vi "cameraTempControllerBackEnd.vi"(8 "error in (no error)":errorcluster, 11 "CameraTempController":refnum<class "CameraTempController.lvclass">) -> (0 "error out":errorcluster, 3 "CameraTempController out":refnum<class "CameraTempController.lvclass">)   [LabVIEW 2011, in "Hardware.lvlib" / "Channels.lvlib" / "CameraTempController.lvclass"]
uses:
  CameraTempController.lvclass
panel:
  in  "tempControllerBackEndEvents":T1
  in  "tempControllerFrontEndEvents":T2
  out "Cooling":bool=TRUE
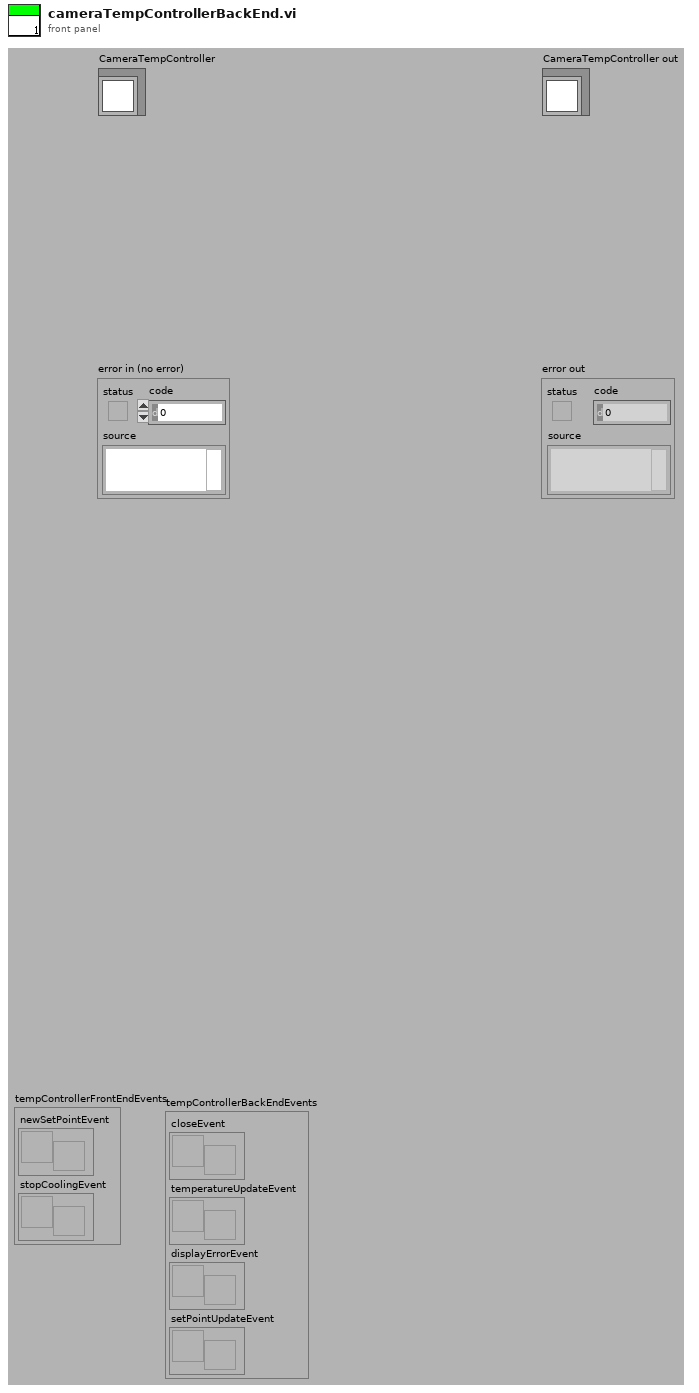
[diagram p1: front panel]
types:
  T1 = cluster{"closeEvent":refnum<user-event>, "temperatureUpdateEvent":refnum<user-event>, "displayErrorEvent":refnum<user-event>, "setPointUpdateEvent":refnum<user-event>}
  T2 = cluster{"newSetPointEvent":refnum<user-event>, "stopCoolingEvent":refnum<user-event>}
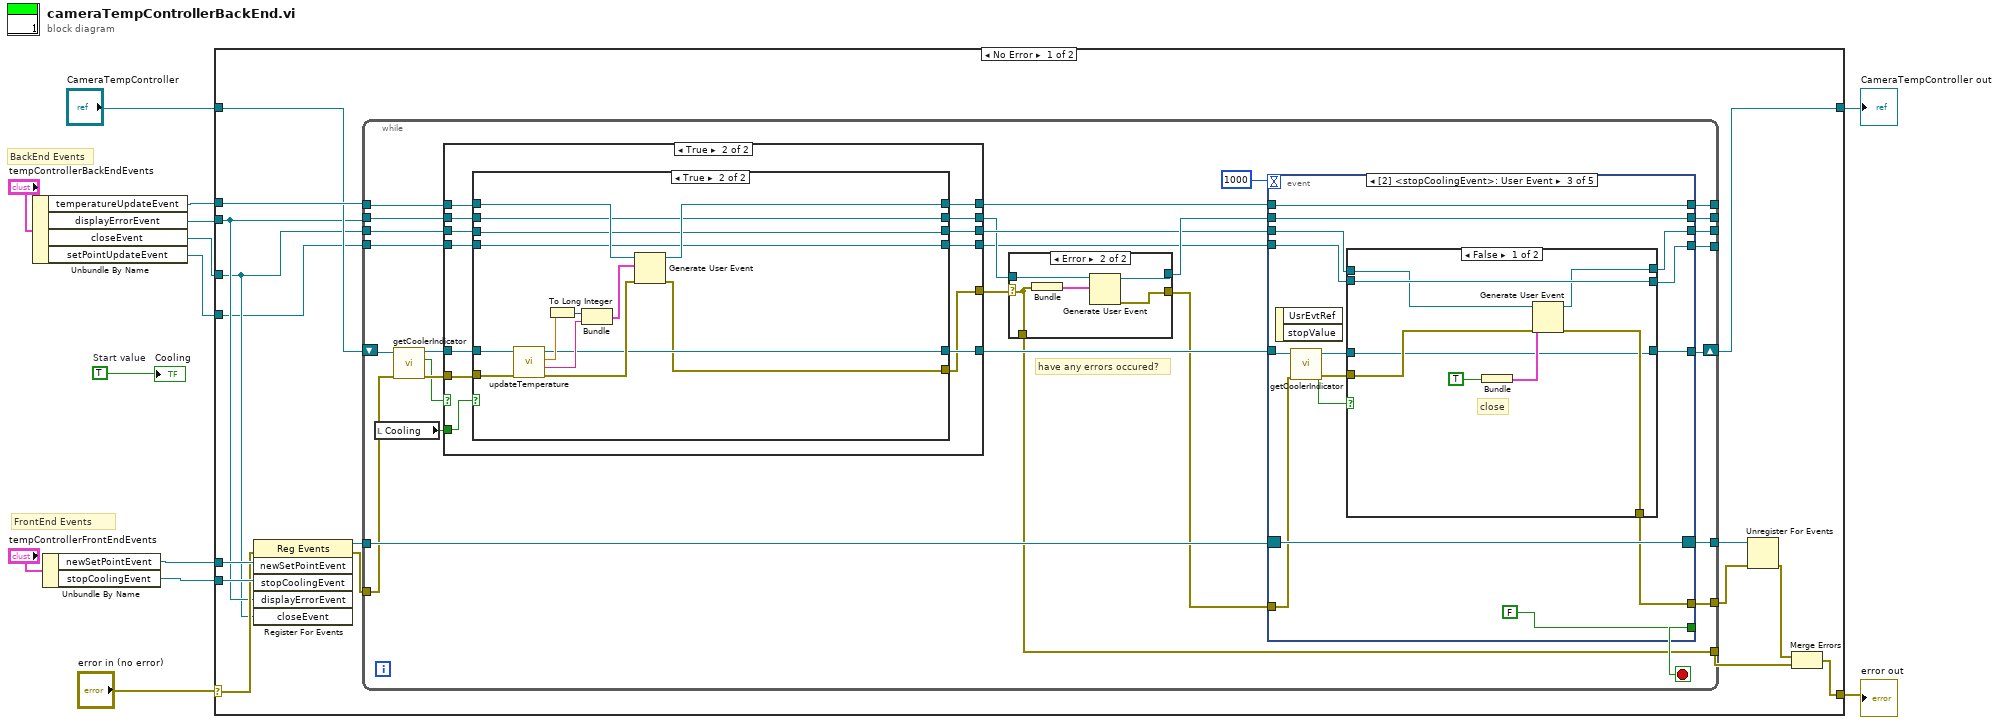
[diagram p0: block diagram]
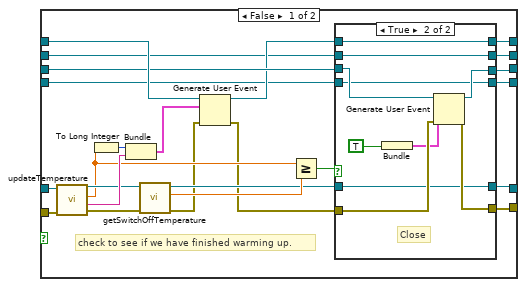
[diagram p3: hidden frame]
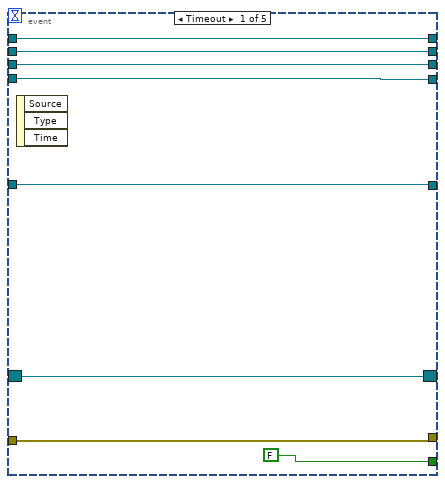
[diagram p6: hidden frame]
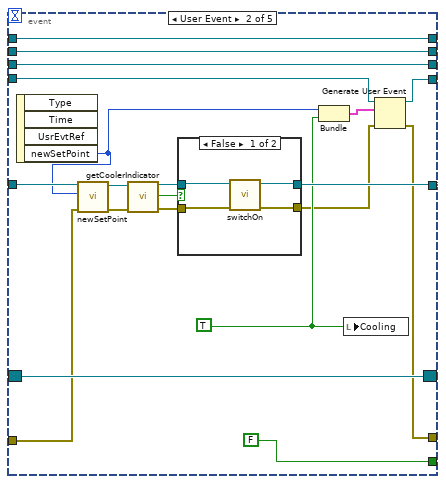
[diagram p7: hidden frame]
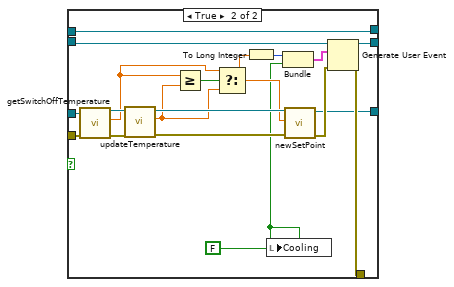
[diagram p9: hidden frame]
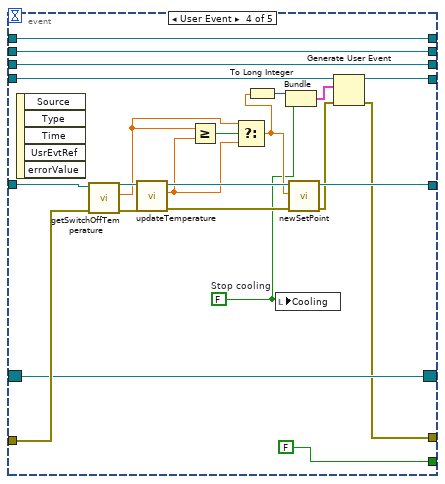
[diagram p10: hidden frame]
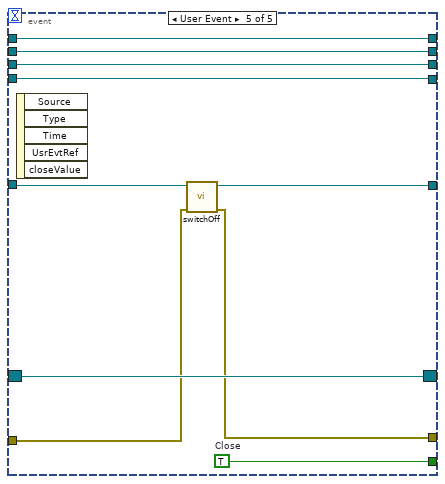
[diagram p11: hidden frame]
diagram:
  w9 = TRUE  # Start value
  # "FrontEnd Events"
  # "BackEnd Events"
  n1 = Unbundle By Name("tempControllerBackEndEvents") -> ("temperatureUpdateEvent"=w4:refnum<user-event>, "displayErrorEvent"=w3:refnum<user-event>, "closeEvent"=w2:refnum<user-event>, "setPointUpdateEvent"=w1:refnum<user-event>)
  n2 = Unbundle By Name("tempControllerFrontEndEvents") -> ("newSetPointEvent"=w5:refnum<user-event>, "stopCoolingEvent"=w6:refnum<user-event>)
  n3 = case shown="No Error" "error in (no error)" {
    selector: "error in (no error)" -> [w27 w249]
    tunnel: [w16 w249] -> w12
    tunnel: [w22 w248] -> w10
    tunnel: "CameraTempController" -> [w24 w248]
    tunnel: w4 -> [w26 _]
    tunnel: w3 -> [w21 _]
    tunnel: w2 -> [w19 _]
    tunnel: w5 -> [w29 _]
    tunnel: w6 -> [w28 _]
    tunnel: w1 -> [w15 _]
    frame No Error {
      n4 = register-events(error in=w27, w29, w28, w21, w19) -> (reference out=w25:refnum<event-registration>, error out=w20:errorcluster)  [unwired: 1 in]
      n5 = while {
        tunnel: w26 -> [w54]
        tunnel: w21 -> [w42]
        tunnel: w19 -> [w44]
        tunnel: w25 -> [w58]
        tunnel: w20 -> [w33]
        tunnel: [w57] -> _
        tunnel: [w56] -> _
        tunnel: [w55] -> w23
        shift-right: [w50] -> w22
        shift-left: w24 -> [w34]
        tunnel: [w52] -> _
        tunnel: [w49] -> w14
        tunnel: [w39] -> w17
        tunnel: w15 -> [w38]
        tunnel: [w36] -> _
        stop <- w40 stop-if-true
        # "have any errors occured?"
        n6 = local read "Cooling"() -> (w45:bool)
        n7 = call-dynamic "getCoolerIndicator.vi"("error in (no error)"=w33, "CameraTempController.lvclass in"=w34) -> ("error out"=w32:errorcluster, "Cooler"=w31:bool, "CameraTempController.lvclass out"=w35:refnum<class "CameraTempController.lvclass">)  [unwired: 7 in]
        n8 = case shown="True" w31 {
          tunnel: w54 -> [w64 w77]
          tunnel: [w64 w76] -> w53
          tunnel: [w61 w75] -> w51
          tunnel: [w59 w74] -> w48
          tunnel: w45 -> [_ w73]
          tunnel: w44 -> [w60 w72]
          tunnel: [w60 w71] -> w43
          tunnel: w42 -> [w62 w70]
          tunnel: [w62 w69] -> w41
          tunnel: w38 -> [w63 w68]
          tunnel: [w63 w67] -> w37
          tunnel: w35 -> [w61 w66]
          tunnel: w32 -> [w59 w65]
          frame False {
          }
          frame True {
            n9 = case shown="True" w73 {
              tunnel: w66 -> [w98 w127]
              tunnel: w77 -> [w99 w126]
              tunnel: [w84 w125] -> w76
              tunnel: w65 -> [w97 w124]
              tunnel: [w86 w123] -> w75
              tunnel: [w87 w122] -> w74
              tunnel: w72 -> [w88 w121]
              tunnel: [w85 w121] -> w71
              tunnel: w70 -> [w82 w120]
              tunnel: [w81 w120] -> w69
              tunnel: w68 -> [w80 w119]
              tunnel: [w79 w119] -> w67
              frame False {
                # "check to see if we have finished warming up."
                n10 = call-dynamic "updateTemperature.vi"("error in (no error)"=w97, "CameraTempController in"=w98) -> ("error out"=w95:errorcluster, "Status"=w101:string, "updateTemperature"=w94:dbl, "CameraTempController out"=w96:refnum<class "CameraTempController.lvclass">)  [unwired: 6 in]
                n11 = To Long Integer(number=w94) -> (32bit integer=w78:i32)
                n12 = Bundle(w78, "Status"=w101) -> (w100:cluster{i32, "Status":string})  [unwired: 1 in]
                n13 = call-dynamic "getSwitchOffTemperature.vi"("error in (no error)"=w95, "CameraTempController in"=w96) -> ("error out"=w90:errorcluster, "Switch Off Temperature"=w93:dbl, "CameraTempController out"=w91:refnum<class "CameraTempController.lvclass">)  [unwired: 7 in]
                n14 = Generate User Event(user event=w99, event data cluster=w100, error in=w90) -> (user event out=w83:refnum<user-event>, error out=w89:errorcluster)
                n15 = Greater Or Equal?(x=w94, y=w93) -> (x >= y?=w92:bool)
                n16 = case shown="True" w92 {
                  tunnel: w91 -> [w107 w114]
                  tunnel: w89 -> [w106 w116]
                  tunnel: w88 -> [w105 w117]
                  tunnel: [w106 w115] -> w87
                  tunnel: [w107 w114] -> w86
                  tunnel: [w105 w113] -> w85
                  tunnel: [w103 w110] -> w84
                  tunnel: w83 -> [w103 w110]
                  tunnel: w82 -> [w104 w109]
                  tunnel: [w104 w109] -> w81
                  tunnel: [w102 w108] -> w79
                  tunnel: w80 -> [w102 w108]
                  frame False {
                  }
                  frame True {
                    # "Close"
                    n17 = Bundle(TRUE) -> (w111:cluster{bool})  [unwired: 1 in]
                    n18 = Generate User Event(user event=w117, event data cluster=w111, error in=w116) -> (user event out=w113:refnum<user-event>, error out=w115:errorcluster)
                  }
                }
              }
              frame True {
                n19 = call-dynamic "updateTemperature.vi"("error in (no error)"=w124, "CameraTempController in"=w127) -> ("error out"=w128:errorcluster, "Status"=w130:string, "updateTemperature"=w131:dbl, "CameraTempController out"=w123:refnum<class "CameraTempController.lvclass">)  [unwired: 6 in]
                n20 = To Long Integer(number=w131) -> (32bit integer=w118:i32)
                n21 = Bundle(w118, "Status"=w130) -> (w129:cluster{i32, "Status":string})  [unwired: 1 in]
                n22 = Generate User Event(user event=w126, event data cluster=w129, error in=w128) -> (user event out=w125:refnum<user-event>, error out=w122:errorcluster)
              }
            }
          }
        }
        n23 = case shown="Error" w48 {
          selector: w48 -> [w132 w134]
          tunnel: [w132 w136] -> w47
          tunnel: w41 -> [w133 w138]
          tunnel: [w133 w135] -> w46
          tunnel: [w132 w134] -> w39
          frame No Error {
          }
          frame Error {
            n24 = Bundle("error IO"=w134) -> (w137:cluster{"error IO":errorcluster})  [unwired: 1 in]
            n25 = Generate User Event(user event=w138, event data cluster=w137) -> (user event out=w135:refnum<user-event>, error out=w136:errorcluster)  [unwired: 1 in]
          }
        }
        n26 = event shown="[2] <stopCoolingEvent>: User Event" {
          selector: w58 -> [w141 w163 w185 w232 w246]
          dyn-events: [w141 w163 w185 w232 w246] -> w55
          timeout: 1000 -> [_ _ _ _ _]
          tunnel: w53 -> [w146 w166 w187 w237 w245]
          tunnel: w46 -> [w145 w165 w186 w236 w244]
          tunnel: w43 -> [w144 w164 w175 w235 w243]
          tunnel: w47 -> [w142 w162 w180 w233 w240]
          tunnel: [w146 w166 w187 w237 w245] -> w52
          tunnel: [w145 w165 w186 w236 w244] -> w57
          tunnel: [w144 w164 w174 w235 w243] -> w56
          tunnel: [w143 w156 w173 w231 w241] -> w50
          tunnel: [w142 w147 w181 w219 w239] -> w49
          tunnel: w51 -> [w143 w155 w179 w234 w242]
          tunnel: [FALSE FALSE FALSE FALSE w247] -> w40
          tunnel: w37 -> [w139 w153 w183 w222 w238]
          tunnel: [w139 w152 w182 w221 w238] -> w36
          event Timeout {
            n27 = event-data() -> ()  [unwired: 1 in, 3 out]
          }
          event User Event {
            w149 = TRUE
            n28 = event-data() -> ("newSetPoint"=w151:i32)  [unwired: 1 in, 3 out]
            n29 = call-dynamic "newSetPoint.vi"("error in (no error)"=w162, "setTemperature"=w151, "CameraTempController in"=w155) -> ("error out"=w160:errorcluster, "CameraTempController out"=w161:refnum<class "CameraTempController.lvclass">)  [unwired: 7 in]
            n30 = call-dynamic "getCoolerIndicator.vi"("error in (no error)"=w160, "CameraTempController.lvclass in"=w161) -> ("error out"=w157:errorcluster, "Cooler"=w159:bool, "CameraTempController.lvclass out"=w158:refnum<class "CameraTempController.lvclass">)  [unwired: 7 in]
            n31 = case shown="False" w159 {
              tunnel: w158 -> [w170 w172]
              tunnel: w157 -> [w169 w171]
              tunnel: [w167 w172] -> w156
              tunnel: [w168 w171] -> w148
              frame False {
                n32 = call-dynamic "switchOn.vi"("error in (no error)"=w169, "CameraTempController in"=w170) -> ("error out"=w168:errorcluster, "CameraTempController out"=w167:refnum<class "CameraTempController.lvclass">)  [unwired: 8 in]
              }
              frame True {
              }
            }
            n33 = Bundle("newSetPoint"=w151, w149) -> (w150:cluster{"newSetPoint":i32, bool})  [unwired: 1 in]
            n34 = local write "Cooling"(w149) -> ()
            n35 = Generate User Event(user event=w153, event data cluster=w150, error in=w148) -> (user event out=w152:refnum<user-event>, error out=w147:errorcluster)
          }
          event User Event {
            n36 = event-data() -> ()  [unwired: 1 in, 2 out]
            n37 = call-dynamic "getCoolerIndicator.vi"("error in (no error)"=w180, "CameraTempController.lvclass in"=w179) -> ("error out"=w176:errorcluster, "Cooler"=w178:bool, "CameraTempController.lvclass out"=w177:refnum<class "CameraTempController.lvclass">)  [unwired: 7 in]
            n38 = case shown="False" w178 {
              tunnel: w183 -> [w193 w207]
              tunnel: [w193 w206] -> w182
              tunnel: [w189 w203] -> w181
              tunnel: w177 -> [w188 w199]
              tunnel: w176 -> [w190 w198]
              tunnel: w175 -> [w192 w197]
              tunnel: [w191 w197] -> w174
              tunnel: [w188 w196] -> w173
              frame False {
                # "close"
                n39 = Bundle(TRUE) -> (w194:cluster{bool})  [unwired: 1 in]
                n40 = Generate User Event(user event=w192, event data cluster=w194, error in=w190) -> (user event out=w191:refnum<user-event>, error out=w189:errorcluster)
              }
              frame True {
                w201 = FALSE
                n41 = call-dynamic "getSwitchOffTemperature.vi"("error in (no error)"=w198, "CameraTempController in"=w199) -> ("error out"=w211:errorcluster, "Switch Off Temperature"=w209:dbl, "CameraTempController out"=w212:refnum<class "CameraTempController.lvclass">)  [unwired: 7 in]
                n42 = call-dynamic "updateTemperature.vi"("error in (no error)"=w211, "CameraTempController in"=w212) -> ("error out"=w214:errorcluster, "updateTemperature"=w208:dbl, "CameraTempController out"=w213:refnum<class "CameraTempController.lvclass">)  [unwired: 6 in, 1 out]
                n43 = Greater Or Equal?(x=w209, y=w208) -> (x >= y?=w210:bool)
                n44 = Select(t=w209, s=w210, f=w208) -> (s? t:f=w202:dbl)
                n45 = To Long Integer(number=w202) -> (32bit integer=w200:i32)
                n46 = local write "Cooling"(w201) -> ()
                n47 = Bundle(w200, w201) -> (w205:cluster{i32, bool})  [unwired: 1 in]
                n48 = call-dynamic "newSetPoint.vi"("error in (no error)"=w214, "setTemperature"=w202, "CameraTempController in"=w213) -> ("error out"=w204:errorcluster, "CameraTempController out"=w196:refnum<class "CameraTempController.lvclass">)  [unwired: 7 in]
                n49 = Generate User Event(user event=w207, event data cluster=w205, error in=w204) -> (user event out=w206:refnum<user-event>, error out=w203:errorcluster)
              }
            }
          }
          event User Event {
            w216 = FALSE  # Stop cooling
            n50 = event-data() -> ()  [unwired: 1 in, 5 out]
            n51 = call-dynamic "getSwitchOffTemperature.vi"("error in (no error)"=w233, "CameraTempController in"=w234) -> ("error out"=w227:errorcluster, "Switch Off Temperature"=w225:dbl, "CameraTempController out"=w228:refnum<class "CameraTempController.lvclass">)  [unwired: 7 in]
            n52 = call-dynamic "updateTemperature.vi"("error in (no error)"=w227, "CameraTempController in"=w228) -> ("error out"=w230:errorcluster, "updateTemperature"=w224:dbl, "CameraTempController out"=w229:refnum<class "CameraTempController.lvclass">)  [unwired: 6 in, 1 out]
            n53 = Greater Or Equal?(x=w225, y=w224) -> (x >= y?=w226:bool)
            n54 = Select(t=w225, s=w226, f=w224) -> (s? t:f=w217:dbl)
            n55 = To Long Integer(number=w217) -> (32bit integer=w215:i32)
            n56 = local write "Cooling"(w216) -> ()
            n57 = Bundle(w215, "Stop cooling"=w216) -> (w218:cluster{i32, "Stop cooling":bool})  [unwired: 1 in]
            n58 = call-dynamic "newSetPoint.vi"("error in (no error)"=w230, "setTemperature"=w217, "CameraTempController in"=w229) -> ("error out"=w220:errorcluster, "CameraTempController out"=w231:refnum<class "CameraTempController.lvclass">)  [unwired: 7 in]
            n59 = Generate User Event(user event=w222, event data cluster=w218, error in=w220) -> (user event out=w221:refnum<user-event>, error out=w219:errorcluster)
          }
          event User Event {
            w247 = TRUE  # Close
            n60 = event-data() -> ()  [unwired: 1 in, 5 out]
            n61 = call-dynamic "switchOff.vi"("error in (no error)"=w240, "CameraTempController in"=w242) -> ("error out"=w239:errorcluster, "CameraTempController out"=w241:refnum<class "CameraTempController.lvclass">)  [unwired: 8 in]
          }
        }
      }
      n62 = Unregister For Events(event registration refnum=w23, error in=w14) -> (error out=w18:errorcluster)
      n63 = Merge Errors(w18, w17) -> (w16:errorcluster)
    }
    frame Error {
    }
  }
  "error out" <- w12
  "CameraTempController out" <- w10
  "Cooling" <- w9
